vi "CMD enabled PI Controller with Stability Checker.vi"(0 "CtrlIndex":i32, 2 "PI Parameters":T1, 5 "Feedback":dbl[](array[numeric]), 9 "CommandCluster":T3, 11 "Stability In":T2, 13 "Tolerances":dbl[](array[numeric])) -> (4 "Output":dbl, 6 "PIdata":dbl[](array[numeric]), 10 "Stable?":bool, 15 "Stability Out":T2)   [LabVIEW 2013]
uses:
  TypeDef/Command Cluster.ctl
  TypeDef/PI Parameters.ctl
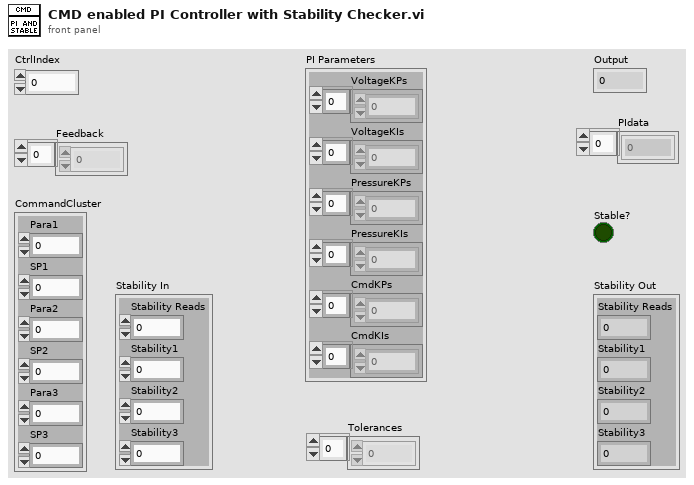
[diagram p1: front panel]
types:
  T1 = typedef "PI Parameters.ctl" = cluster{"VoltageKPs":dbl[], "VoltageKIs":dbl[], "PressureKPs":dbl[], "PressureKIs":dbl[], "CmdKPs":dbl[], "CmdKIs":dbl[]}
  T2 = cluster{"Stability Reads":i32, "Stability1":i32, "Stability2":i32, "Stability3":i32}
  T3 = typedef "Command Cluster.ctl" = cluster{"Para1":i32, "SP1":dbl, "Para2":i32, "SP2":dbl, "Para3":i32, "SP3":dbl}
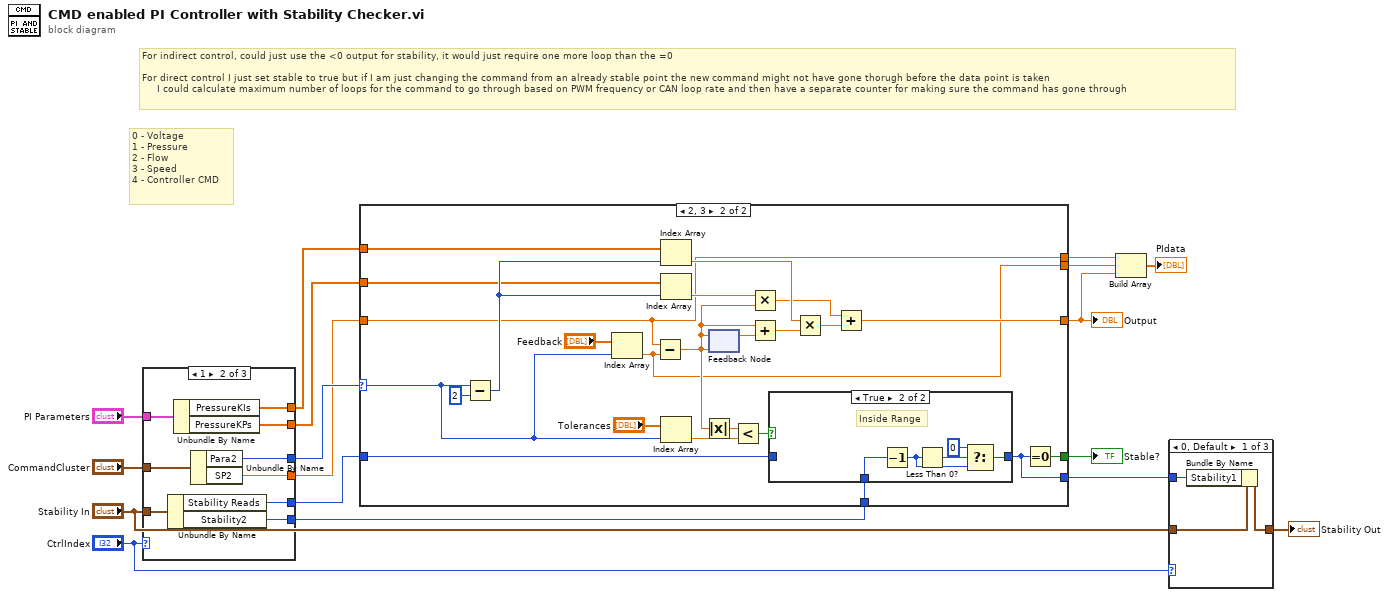
[diagram p0: block diagram]
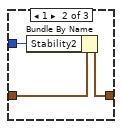
[diagram p2: hidden frame]
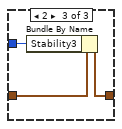
[diagram p3: hidden frame]
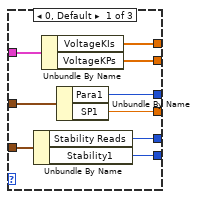
[diagram p4: hidden frame]
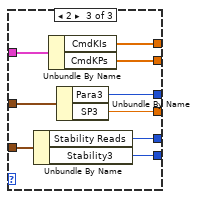
[diagram p5: hidden frame]
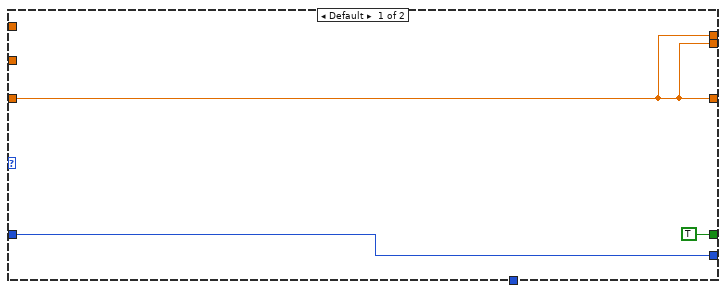
[diagram p6: hidden frame]
diagram:
  # "For indirect control, could just use the <0 output for stability, it would just require one more loop than the =0\n\nFor direct control I just set stable to true but if I am just changing the command from an already stable point the new command might not have gone thorugh before the data point is taken\n     I could calculate maximum number of loops for the command to go through based on PWM frequency or CAN loop rate and then have a separate counter for making sure the command has gone through"
  # "0 - Voltage\n1 - Pressure\n2 - Flow\n3 - Speed\n4 - Controller CMD"
  n1 = case shown="1" "CtrlIndex" {
    tunnel: "Stability In" -> [w26 w35 w44]
    tunnel: [w24 w33 w42] -> w15
    tunnel: [w25 w34 w43] -> w12
    tunnel: "CommandCluster" -> [w23 w32 w41]
    tunnel: [w22 w31 w40] -> w14
    tunnel: [w21 w30 w39] -> w13
    tunnel: "PI Parameters" -> [w18 w29 w38]
    tunnel: [w20 w28 w37] -> w6
    tunnel: [w19 w27 w36] -> w5
    frame 0, Default {
      n2 = Unbundle By Name(w26) -> ("Stability Reads"=w24:i32, "Stability1"=w25:i32)
      n3 = Unbundle By Name(w18) -> ("VoltageKIs"=w20:dbl[], "VoltageKPs"=w19:dbl[])
      n4 = Unbundle By Name(w23) -> ("Para1"=w22:i32, "SP1"=w21:dbl)
    }
    frame 1 {
      n5 = Unbundle By Name(w35) -> ("Stability Reads"=w33:i32, "Stability2"=w34:i32)
      n6 = Unbundle By Name(w29) -> ("PressureKIs"=w28:dbl[], "PressureKPs"=w27:dbl[])
      n7 = Unbundle By Name(w32) -> ("Para2"=w31:i32, "SP2"=w30:dbl)
    }
    frame 2 {
      n8 = Unbundle By Name(w44) -> ("Stability Reads"=w42:i32, "Stability3"=w43:i32)
      n9 = Unbundle By Name(w38) -> ("CmdKIs"=w37:dbl[], "CmdKPs"=w36:dbl[])
      n10 = Unbundle By Name(w41) -> ("Para3"=w40:i32, "SP3"=w39:dbl)
    }
  }
  n11 = case shown="2, 3" w14 {
    selector: w14 -> [_ w52]
    tunnel: w13 -> [w45 w48]
    tunnel: [w45 w58] -> w4
    tunnel: [TRUE w57] -> w17
    tunnel: [w47 w56] -> w8
    tunnel: w15 -> [w47 w55]
    tunnel: w12 -> [_ w54]
    tunnel: w6 -> [_ w51]
    tunnel: w5 -> [_ w50]
    tunnel: [w45 w49] -> w3
    tunnel: [w45 w48] -> w2
    frame Default {
    }
    frame 2, 3 {
      n12 = Subtract(x=w52, y=2) -> (x-y=w59:i32)
      n13 = Index Array(array="Feedback", index=w52) -> (element=w49:dbl)
      n14 = Subtract(x=w48, y=w49) -> (x-y=w69:dbl)
      n15 = Index Array(array=w51, index=w59) -> (element=w65:dbl)
      n16 = Index Array(array=w50, index=w59) -> (element=w63:dbl)
      n17 = Index Array(array="Tolerances", index=w52) -> (element=w60:dbl)
      n18 = Absolute Value(x=w69) -> (abs(x)=w61:dbl)
      n19 = feedback #1(w69) -> (w68:dbl)
      n20 = feedback-in #1(w69) -> ()
      n21 = Less?(x=w61, y=w60) -> (x < y?=w62:bool)
      n22 = Multiply(x=w63, y=w69) -> (x*y=w64:dbl)
      n23 = Add(x=w69, y=w68) -> (x+y=w67:dbl)
      n24 = case shown="True" w62 {
        tunnel: [w72 w74] -> w56
        tunnel: w55 -> [w72 _]
        tunnel: w54 -> [_ w73]
        frame False {
          # "Outside Range"
        }
        frame True {
          # "Inside Range"
          n25 = Decrement(x=w73) -> (x-1=w76:i32)
          n26 = Less Than 0?(x=w76) -> (x < 0?=w75:bool)
          n27 = Select(t=0, s=w75, f=w76) -> (s? t:f=w74:i32)
        }
      }
      n28 = Multiply(x=w65, y=w67) -> (x*y=w66:dbl)
      n29 = Add(x=w64, y=w66) -> (x+y=w58:dbl)
      n30 = Equal To 0?(x=w56) -> (x = 0?=w57:bool)
    }
  }
  "Output" <- w4
  "Stable?" <- w17
  n31 = Build Array(w2, w3, w4) -> (→"PIdata":dbl[])
  n32 = case shown="0, Default" "CtrlIndex" {
    tunnel: "Stability In" -> [w79 w82 w85]
    tunnel: [w78 w81 w84] -> w11
    tunnel: w8 -> [w80 w83 w86]
    frame 0, Default {
      n33 = Bundle By Name(cluster=w79, "Stability1"=w80) -> (w78:T2)
    }
    frame 1 {
      n34 = Bundle By Name(cluster=w82, "Stability2"=w83) -> (w81:T2)
    }
    frame 2 {
      n35 = Bundle By Name(cluster=w85, "Stability3"=w86) -> (w84:T2)
    }
  }
  "Stability Out" <- w11
